vi "parse_results_for_max_v2.vi"(11 "input file":path=path "C:/Users/hpDIRC/Desktop/260508testsIR_1-3.csv") -> (3 "max-only path":path)   [LabVIEW 2024]
uses:
  c718c117-2af1-4f26-a2c0-073317b5ceac.vi
  3bac7da3-b819-48ca-ac31-15608745786e.vi
panel:
  out "spreadsheet string":string
  out "MAX ONLY":string[][](array[string])
  out "meas#":string[](array[string])
  out "bar-notes":string[](array[string])
  out "text":string
  out "error out":errorcluster
  # "0 time\n1 pd1\n2 pd2\n3 pd3\n4 pd3/pd1\n5 pd2/pd1\n6 bx\n7 by\n8 pdx\n9 pdy\n10 pda\n11 bm\n12 bar-note\n13 meas#\n14 pt#\n15 Temp"
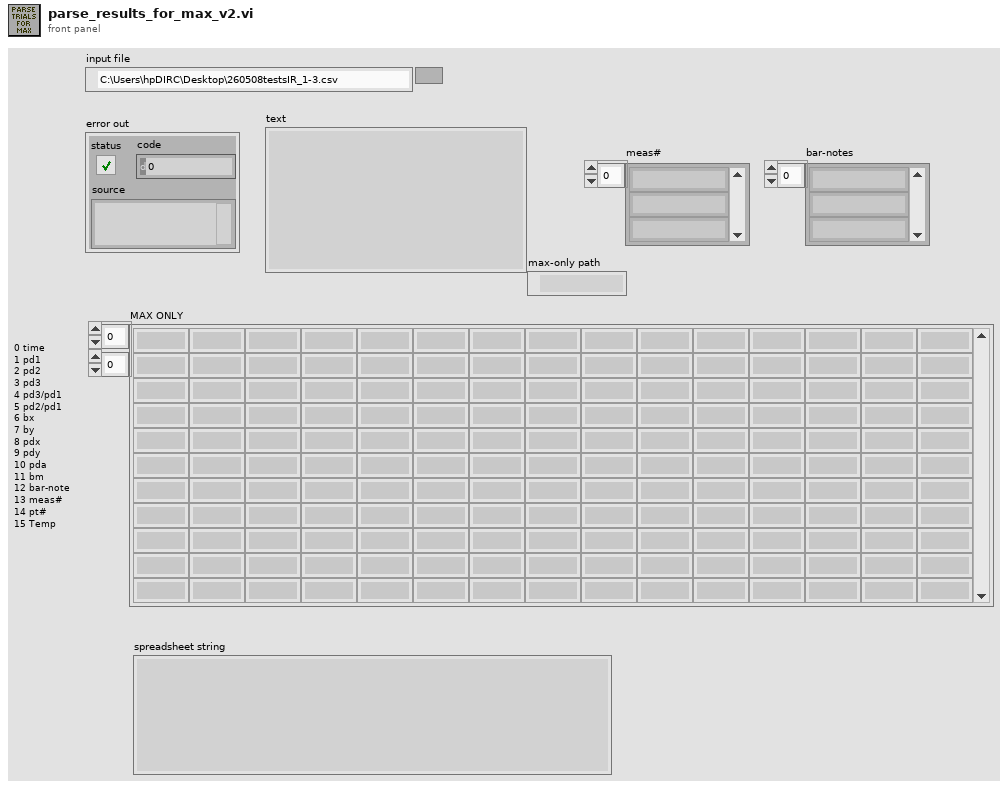
[diagram p1: front panel]
types:
  T1 = enum16{"open", "replace", "create", "open or create", "replace or create", "replace or create with confirmation"}
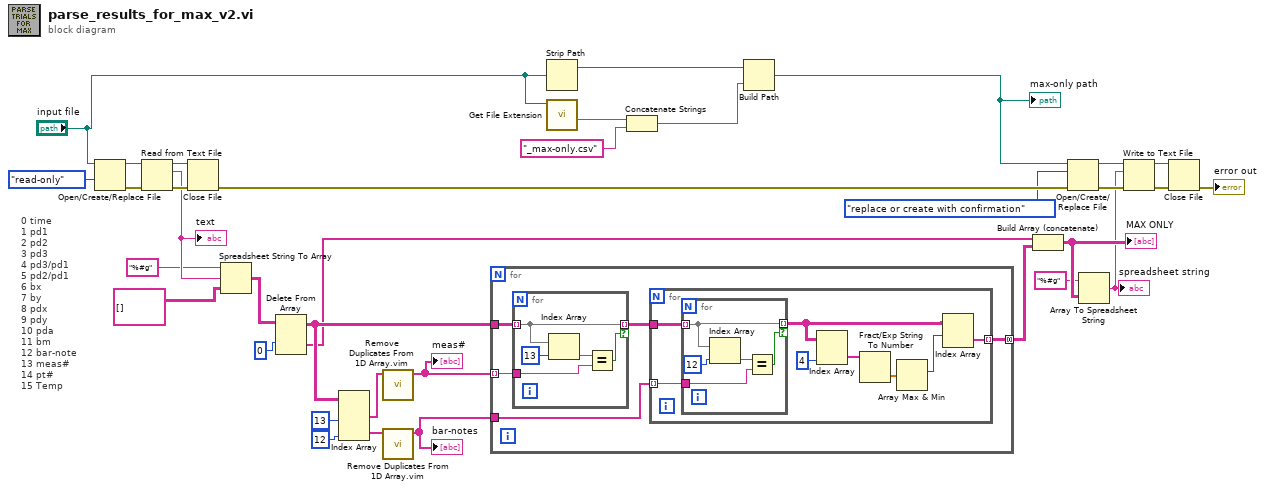
[diagram p0: block diagram]
diagram:
  # "0 time\n1 pd1\n2 pd2\n3 pd3\n4 pd3/pd1\n5 pd2/pd1\n6 bx\n7 by\n8 pdx\n9 pdy\n10 pda\n11 bm\n12 bar-note\n13 meas#\n14 pt#\n15 Temp"
  n1 = Open/Create/Replace File(file path (use dialog)="input file", access (0:read/write)=enum16{"read/write", "read-only", "write-only"}."read-only") -> (refnum out=w35:refnum<file>, error out=w34:errorcluster)  [unwired: 4 in, 1 out]
  n2 = Read from Text File(file (use dialog)=w35, error in=w34) -> (refnum out=w32:refnum<file>, text=w31:string, error out=w33:errorcluster)  [unwired: 2 in, 1 out]
  "text" <- w31
  n3 = Close File(refnum=w32, error in=w33) -> (error out=w13:errorcluster)  [unwired: 1 out]
  n4 = Spreadsheet String To Array(format string="%#g", spreadsheet string=w31, array type (2D Dbl)=string[][] []) -> (array=w28:string[][])  [unwired: 1 in]
  n5 = Delete From Array(array=w28, index (row)=0 ("disabled index (col)")) -> (deleted portion=w19:string[], array with subset deleted=w25:string[][])  [unwired: 2 in]
  n6 = Index Array(array=w25, index (col) #1=13 ("index (col)"), index (col) #2=12 ("index (col)")) -> (element #1=w22:string[], element #2=w20:string[])  [unwired: 2 in]
  n7 = call "Remove Duplicates From 1D Array.vim"("array"=w22) -> ("array with duplicates removed"=w26:string[])  [unwired: 10 in]
  "meas#" <- w26
  n8 = call "Remove Duplicates From 1D Array.vim"("array"=w20) -> ("array with duplicates removed"=w24:string[])  [unwired: 10 in]
  "bar-notes" <- w24
  n9 = for {
    tunnel: w25 -> [w40]
    tunnel: w26 -> [w39] mode=indexing
    tunnel: w24 -> [w38]
    tunnel: [w36] -> w18 mode=concatenating
    n10 = for {
      tunnel: w40 -> [w55] mode=indexing
      tunnel: w39 -> [w56]
      tunnel: [w55] -> w37 mode=indexing if=w54
      n11 = Index Array(array=w55, index=13) -> (element=w57:string)
      n12 = Equal?(x=w57, y=w56) -> (x = y?=w54:bool)
    }
    n13 = for {
      tunnel: w38 -> [w47] mode=indexing
      tunnel: w37 -> [w48]
      tunnel: [w41] -> w36 mode=indexing
      n14 = for {
        tunnel: w48 -> [w50] mode=indexing
        tunnel: w47 -> [w51]
        tunnel: [w50] -> w43 mode=indexing if=w49
        n15 = Index Array(array=w50, index=12) -> (element=w52:string)
        n16 = Equal?(x=w52, y=w51) -> (x = y?=w49:bool)
      }
      n17 = Index Array(array=w43, index (col)=4 ("disabled index (col)")) -> (element=w45:string[])  [unwired: 1 in]
      n18 = Fract/Exp String To Number(string=w45) -> (number=w44:dbl[])  [unwired: 3 in, 1 out]
      n19 = Array Max & Min(array=w44) -> (max index (indices)=w42:i32)  [unwired: 3 out]
      n20 = Index Array(array=w43, index (row)=w42) -> (element=w41:string[])  [unwired: 1 in]
    }
  }
  n21 = Strip Path(path="input file") -> (stripped path=w4:path)  [unwired: 1 out]
  n22 = call <vilib>:"Get File Extension.vi"("file"="input file") -> ("filename without extension"=w6:string)  [unwired: 6 in, 4 out]
  n23 = Concatenate Strings(w6, "_max-only.csv" ("string")) -> (w3:string)
  n24 = Build Path(base path=w4, name or relative path=w3) -> (appended path=w2:path)
  "max-only path" <- w2
  n25 = Build Array (concatenate)(w19, w18) -> (w17:string[][])
  "MAX ONLY" <- w17
  n26 = Open/Create/Replace File(file path (use dialog)=w2, error in=w13, operation (0:open)=T1."replace or create with confirmation") -> (refnum out=w10:refnum<file>, error out=w15:errorcluster)  [unwired: 3 in, 1 out]
  n27 = Array To Spreadsheet String(array=w17, 3:"%#g" ("format string")) -> (spreadsheet string=w11:string)  [unwired: 1 in]
  "spreadsheet string" <- w11
  n28 = Write to Text File(file (use dialog)=w10, text=w11, error in=w15) -> (refnum out=w9:refnum<file>, error out=w14:errorcluster)  [unwired: 1 in, 1 out]
  n29 = Close File(refnum=w9, error in=w14) -> (error out=→"error out":errorcluster)  [unwired: 1 out]
